vi "Set Status Source.vi"(8 "error in (no error)":errorcluster, 10 "Status Source":T1, 11 "VISA resource name in":refnum<visa-resource-name>) -> (0 "error out":errorcluster, 3 "VISA resource name":refnum<visa-resource-name>)   [LabVIEW 2023, in "CTI-Visa.lvlib"]
uses:
  CTI-Visa.lvlib
  Status Source.ctl
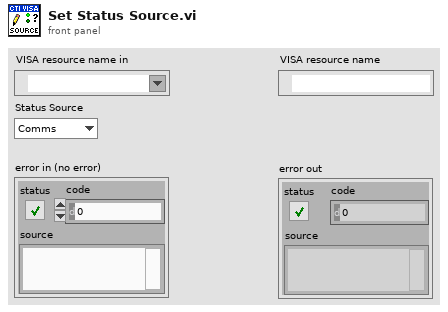
[diagram p1: front panel]
types:
  T1 = typedef "CTI-Visa.lvlib/Status Source.ctl" = enum16{"Comms", "User"}
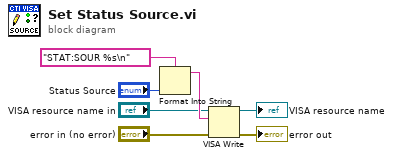
[diagram p0: block diagram]
diagram:
  n1 = Format Into String(format string="STAT:SOUR %s\n", "Status Source") -> (resulting string=w7:string)  [unwired: 2 in, 1 out]
  n2 = VISA Write(VISA resource name="VISA resource name in", write buffer=w7, error in (no error)="error in (no error)") -> (VISA resource name out=→"VISA resource name":refnum<visa-resource-name>, error out=→"error out":errorcluster)  [unwired: 1 out]
